vi "Get Maximum Binning.vi"(8 "error in (no error)":errorcluster, 9 "MaxBinning":i32, 10 "HorzVert":i32, 11 "ReadMode":i32) -> (0 "error out":errorcluster, 1 "MaxBinning out":i32, 3 "function return":u32)   [LabVIEW 2014, in "atmcd32d.lvlib"]
doc: "unsigned int WINAPI GetMaximumBinning(int ReadMode, int HorzVert, int * MaxBinning);"
uses:
  atmcd32d.lvlib
  atmcd32d.dll
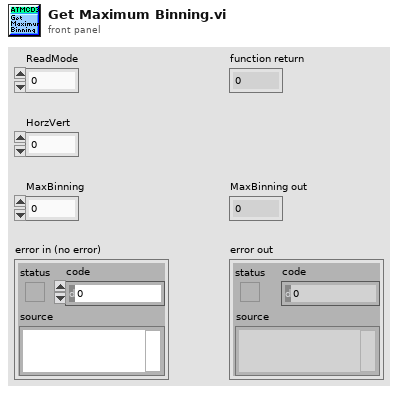
[diagram p1: front panel]
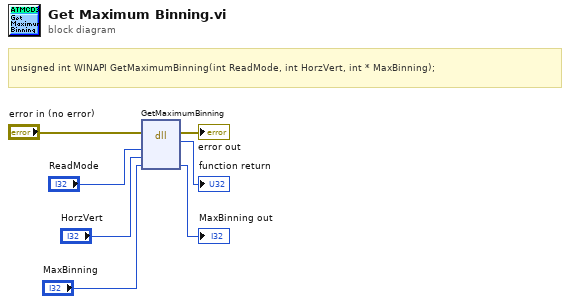
[diagram p0: block diagram]
diagram:
  # "unsigned int WINAPI GetMaximumBinning(int ReadMode, int HorzVert, int * MaxBinning);"
  n1 = dll-call lib="C:/Users/Bakir/Documents/Lambda2-Testing/lib/Andorlib/atmcd32d.*" fn="GetMaximumBinning"(error in="error in (no error)", "ReadMode"="ReadMode", "HorzVert"="HorzVert", "MaxBinning"="MaxBinning") -> (error out=→"error out":errorcluster, →"function return":u32, "MaxBinning"=→"MaxBinning out":i32)  [unwired: 4 in, 1 out]
